vi "SetGetPowerLock.vi"() -> ()   [LabVIEW 2017]
panel:
  out "Out  2":bool
  in  "ES_BOOL":bool
  out "error out":errorcluster
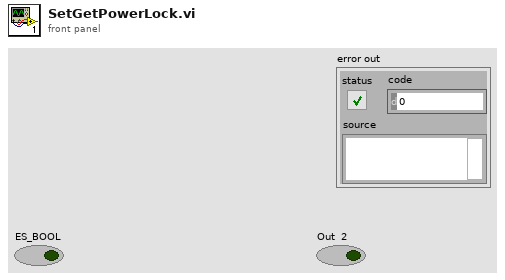
[diagram p1: front panel]
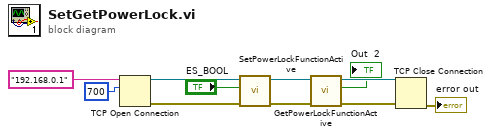
[diagram p0: block diagram]
diagram:
  n1 = TCP Open Connection(address="192.168.0.1", remote port or service name=u16 700) -> (connection ID=w3:refnum<k5>, error out=w4:errorcluster)  [unwired: 3 in]
  n2 = call "SetPowerLockFunctionActive.vi"("error in (no error)"=w4, "ES_BOOL"="ES_BOOL", "TCP Network Connection in"=w3) -> ("error out"=w5:errorcluster, "TCP Network Connection out"=w8:refnum<k5>)  [unwired: 5 in, 2 out]
  n3 = call "GetPowerLockFunctionActive.vi"("error in (no error)"=w5, "TCP Network Connection in"=w8) -> ("error out"=w6:errorcluster, "ES_BOOL"=→"Out  2":bool, "TCP Network Connection out"=w7:refnum<k5>)  [unwired: 5 in, 2 out]
  n4 = TCP Close Connection(connection ID=w7, error in (no error)=w6) -> (error out=→"error out":errorcluster)  [unwired: 1 in, 1 out]
